vi "Do.vi"(8 "error in (no error)":errorcluster, 10 "Actor in":refnum<class "Actor.lvclass">, 11 "WebSocket Service Enqueuer Msg":refnum<class "WebSocket Service Enqueuer Msg.lvclass">) -> (0 "error out":errorcluster, 2 "Actor out":refnum<class "Actor.lvclass">)   [LabVIEW 2021, in "Echo Broadcast With Server Manager.lvlib" / "WebSocket Service Enqueuer Msg.lvclass"]
doc: "(<B>Filename</B>: Actor Framework.lvlib:Message.lvclass:Do.vi)\n\nDefines what a message does when it is received by an actor. Generally, a message instructs an actor to invoke one of its methods. By default, this method does nothing. A child class must override it to define behavior. Create a child class by using the Actor Framework Message Maker dialog box."
uses:
  WebSocket Service Enqueuer Msg.lvclass
  C:/Projects/WebSocket-Actor/WebSocket Actor/Abstract Messages/WebSocket Server-Service Enqueuer Msg/WebSocket Server-Service Enqueuer Msg.lvclass
  <vilib>/ActorFramework/Actor/Actor.lvclass
  WS Test Server Subscriber/WS Test Server Subscriber.lvclass
  C:/Program Files/National Instruments/LabVIEW 2021/vi.lib/ActorFramework/Actor/Actor.lvclass
  WebSocket Actor/Abstract Messages/WebSocket Server-Service Enqueuer Msg/WebSocket Server-Service Enqueuer Msg.lvclass/WebSocket Server-Service Enqueuer Msg.ctl
  WS Test Server Subscriber/WS Test Server Subscriber.lvclass/WS Test Server Subscriber.ctl
  WS Test Server Subscriber/properties/Write WebSocket Service Enqueuer.vi
  WebSocket Actor/Abstract Messages/WebSocket Server-Service Enqueuer Msg/properties/Read WebSocket Service Enqueuer.vi
  <vilib>/ActorFramework/Message Enqueuer/Message Enqueuer.lvclass
  WebSocket Service Enqueuer Msg.lvclass/WebSocket Service Enqueuer Msg.ctl
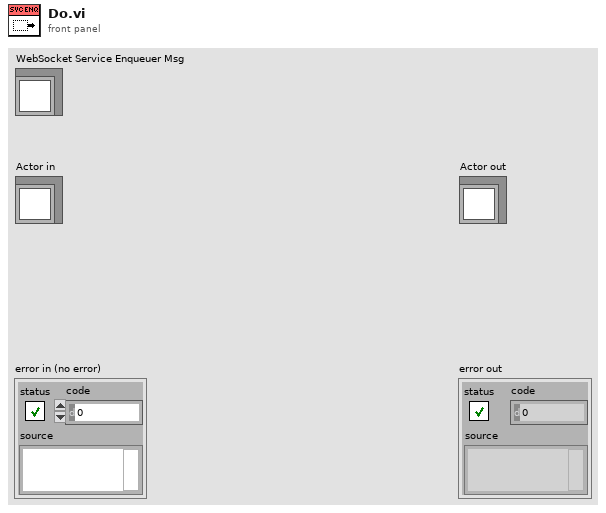
[diagram p1: front panel]
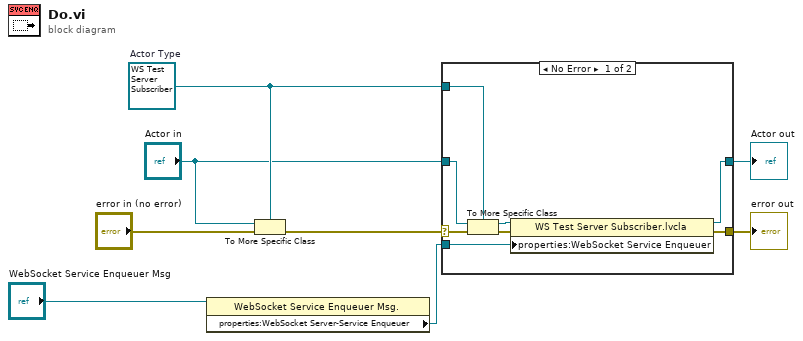
[diagram p0: block diagram]
diagram:
  w7 = refnum<class "WS Test Server Subscriber.lvclass"> refnum  # Actor Type
  n1 = property class="WebSocket Service Enqueuer Msg."(reference="WebSocket Service Enqueuer Msg") -> ("properties:WebSocket Server-Service Enqueuer"=w1:refnum<class "Message Enqueuer.lvclass">)  [unwired: 1 in, 2 out]
  n2 = To More Specific Class(target class=w7, reference="Actor in", error in="error in (no error)") -> (error out=w8:errorcluster)  [unwired: 1 out]
  n3 = case shown="No Error" w8 {
    selector: w8 -> [w16 w18]
    tunnel: [w11 w18] -> w3
    tunnel: [w10 w17] -> w4
    tunnel: "Actor in" -> [w15 w17]
    tunnel: w7 -> [w14 _]
    tunnel: w1 -> [w9 _]
    frame No Error {
      n4 = To More Specific Class ("Actor Cast")(target class=w14, reference=w15, error in=w16) -> (specific class reference=w13:refnum<class "WS Test Server Subscriber.lvclass">, error out=w12:errorcluster)
      n5 = property class="WS Test Server Subscriber.lvcla"(reference=w13, error in=w12, "properties:WebSocket Service Enqueuer"=w9) -> (reference out=w10:refnum<class "WS Test Server Subscriber.lvclass">, error out=w11:errorcluster)
    }
    frame Error {
    }
  }
  "error out" <- w3
  "Actor out" <- w4
